vi "IT8800-Request.vi"(6 "Response?":bool, 8 "error in":errorcluster, 9 "byte count":u32, 10 "Command":string, 11 "IT8800 Setting In In":T1={"VISA Resource Name"="", "Baud Rate"=19200, "Stop Bits"=20, "Wait For Read(ms)"=0} {"Stop Bits" items=["1.0"=10, "2.0"=20]; "Baud Rate" items=["2400"=2400, "4800"=4800, "9600"=9600, "19200"=19200]}) -> (0 "error out":errorcluster, 2 "Response":string, 3 "IT8800 Setting In Out":T1={"VISA Resource Name"="", "Baud Rate"=19200, "Stop Bits"=20, "Wait For Read(ms)"=0} {"Stop Bits" items=["1.0"=10, "2.0"=20]; "Baud Rate" items=["2400"=2400, "4800"=4800, "9600"=9600, "19200"=19200]})   [LabVIEW 2018]
uses:
  Data Def/IT8800-Setting.ctl
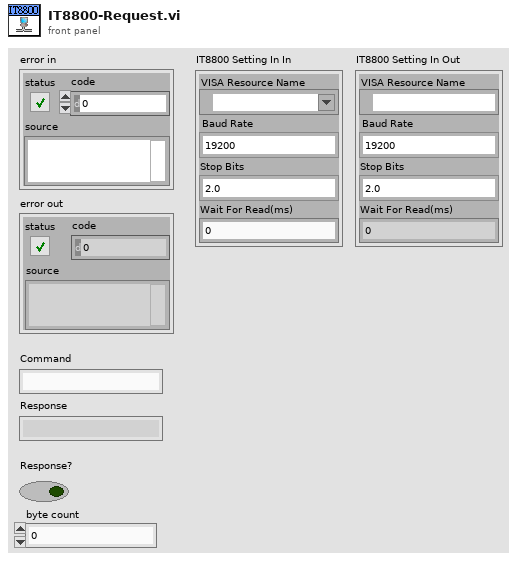
[diagram p1: front panel]
types:
  T1 = typedef "IT8800-Setting.ctl" = cluster{"VISA Resource Name":refnum<visa-resource-name>, "Baud Rate":u32, "Stop Bits":u16, "Wait For Read(ms)":u32}
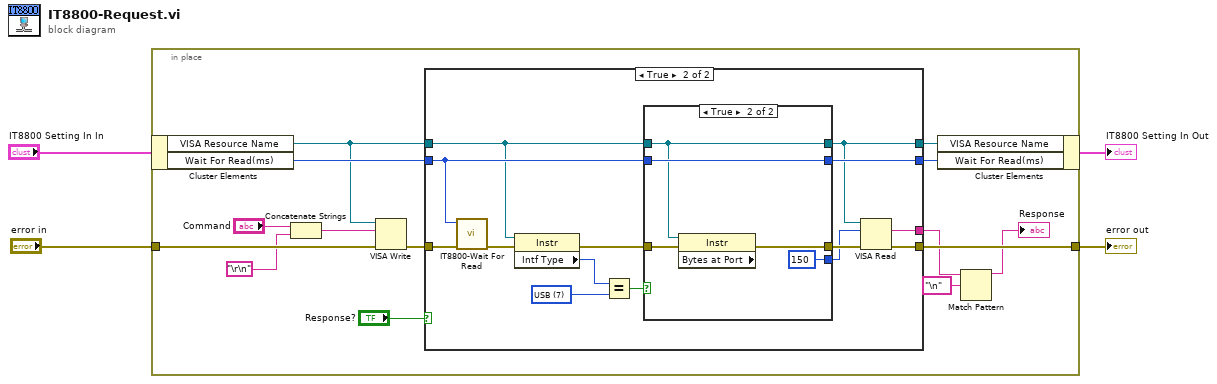
[diagram p0: block diagram]
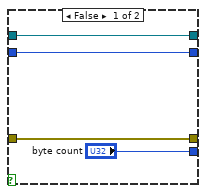
[diagram p3: hidden frame]
diagram:
  n1 = in-place {
    in-place-border: "error in" -> [w18]
    in-place-border: [w15] -> w3
    n2 = in-place-cluster #1("IT8800 Setting In In") -> ("VISA Resource Name"=w13:refnum<visa-resource-name>, "Wait For Read(ms)"=w14:u32)
    n3 = Concatenate Strings("Command", "\r\n") -> (w9:string)
    n4 = VISA Write(VISA resource name=w13, write buffer=w9, error in (no error)=w18) -> (error out=w17:errorcluster)  [unwired: 2 out]
    n5 = case shown="True" "Response?" {
      tunnel: w17 -> [w21 w35]
      tunnel: [w21 w34] -> w15
      tunnel: w13 -> [w19 w25]
      tunnel: w14 -> [w20 w26]
      tunnel: [w19 w22] -> w12
      tunnel: [w20 w24] -> w11
      tunnel: [_ w23] -> w7
      frame False {
      }
      frame True {
        w32 = u16 7 items=["GPIB"=1, "VXI"=2, "GPIB-VXI"=3, "Serial"=4, "PXI"=5, "TCPIP"=6, "USB"=7] ("Interface Information:Interface Type")
        n6 = call "IT8800-Wait For Read.vi"("error in"=w35, "Wait For Read(ms)"=w26) -> ("error out"=w33:errorcluster)  [unwired: 9 in]
        n7 = property class="Instr"(reference=w25, error in=w33) -> (error out=w29:errorcluster, "Intf Type"=w31:u16)  [unwired: 1 out]
        n8 = Equal?(x=w31, y=w32) -> (x = y?=w30:bool)
        n9 = case shown="True" w30 {
          tunnel: w29 -> [w39 w44]
          tunnel: [w39 w43] -> w28
          tunnel: ["byte count" u32 150 ("byte count")] -> w27
          tunnel: w26 -> [w36 w42]
          tunnel: w25 -> [w37 w41]
          tunnel: [w36 w42] -> w24
          tunnel: [w37 w41] -> w22
          frame False {
          }
          frame True {
            n10 = property class="Instr" props=["Bytes at Port"](reference=w41, error in=w44) -> (error out=w43:errorcluster)  [unwired: 2 out]
          }
        }
        n11 = VISA Read(VISA resource name=w22, byte count=w27, error in (no error)=w28) -> (read buffer=w23:string, error out=w34:errorcluster)  [unwired: 2 out]
      }
    }
    n12 = in-place-cluster #1("VISA Resource Name"=w12, "Wait For Read(ms)"=w11) -> (→"IT8800 Setting In Out":T1)
    n13 = Match Pattern(string=w7, regular expression="\n") -> (before substring=→"Response":string)  [unwired: 1 in, 3 out]
  }
  "error out" <- w3
